vi "DSF.Shared.Configuration.Cycle Timed.Initialize.vi"(6 "Cycle Timing Factors":T1={"Decimation"=1, "Offset"=0}, 7 "Custom Parameters":variant, 8 "error in (no error)":errorcluster, 9 "Priority":u8, 10 "Name":string, 11 "Cycle Timed Configuration in":refnum<class "DSF.Shared.Configuration.Cycle Timed.lvclass">) -> (0 "error out":errorcluster, 3 "Cycle Timed Configuration out":refnum<class "DSF.Shared.Configuration.Cycle Timed.lvclass">)   [LabVIEW 2016, in "DSF.Shared.lvlib" / "DSF.Shared.Configuration.Cycle Timed.lvclass"]
uses:
  DSF.Shared.Configuration.Cycle Timed.lvclass
  C:/Git/Sourcetree/DSF/Source/Shared/Classes/Configuration/DSF.Shared.Configuration.lvclass
  Typedefs/DSF.Shared.Typedefs.Cycle Timing Factors.ctl
  DSF.Shared.Configuration.Cycle Timed.lvclass/DSF.Shared.Configuration.Cycle Timed.ctl
  DSF.Shared.Configuration.lvclass
  DSF.Shared.lvlib
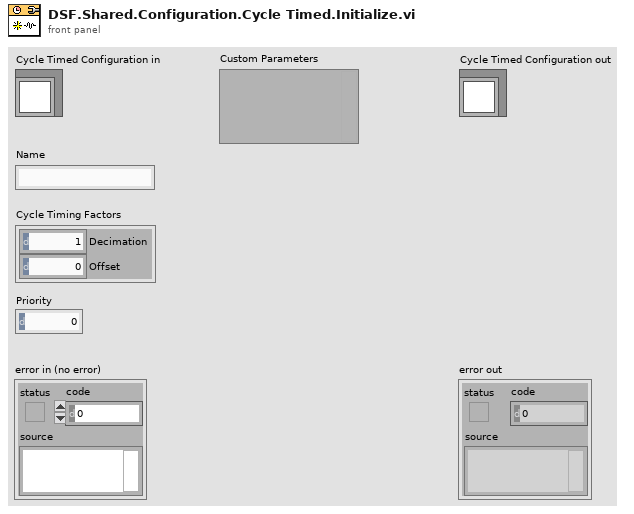
[diagram p1: front panel]
types:
  T1 = typedef "DSF.Shared.lvlib/DSF.Shared.Typedefs.Cycle Timing Factors.ctl" = cluster{"Decimation":u64, "Offset":u64}
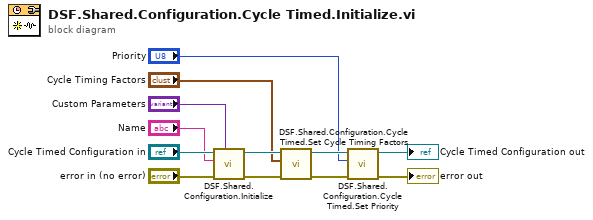
[diagram p0: block diagram]
diagram:
  n1 = call "DSF.Shared.Configuration.Initialize.vi"("Custom Parameters"="Custom Parameters", "error in (no error)"="error in (no error)", "Name"="Name", "Configuration in"="Cycle Timed Configuration in") -> ("error out"=w9:errorcluster, "Configuration out"=w10:refnum<class "DSF.Shared.Configuration.Cycle Timed.lvclass">)  [unwired: 6 in]
  n2 = call "DSF.Shared.Configuration.Cycle Timed.Set Cycle Timing Factors.vi"("error in (no error)"=w9, "Cycle Timing Factors"="Cycle Timing Factors", "Cycle Timed Configuration in"=w10) -> ("error out"=w4:errorcluster, "Cycle Timed Configuration out"=w5:refnum<class "DSF.Shared.Configuration.Cycle Timed.lvclass">)  [unwired: 7 in]
  n3 = call "DSF.Shared.Configuration.Cycle Timed.Set Priority.vi"("error in (no error)"=w4, "Priority"="Priority", "Cycle Timed Configuration in"=w5) -> ("error out"=→"error out":errorcluster, "Cycle Timed Configuration out"=→"Cycle Timed Configuration out":refnum<class "DSF.Shared.Configuration.Cycle Timed.lvclass">)  [unwired: 7 in]
